vi "Static Read.vi"(8 "error in (no error)":errorcluster, 11 "Abs_I16 Integer in":refnum<class "Abs_I16 Integer.lvclass">) -> (0 "error out":errorcluster, 2 "Value":i16, 3 "Abs_I16 Integer out":refnum<class "Abs_I16 Integer.lvclass">)   [LabVIEW 2021, in "Abs_I16 Integer.lvclass"]
uses:
  Abs_I16 Integer.lvclass
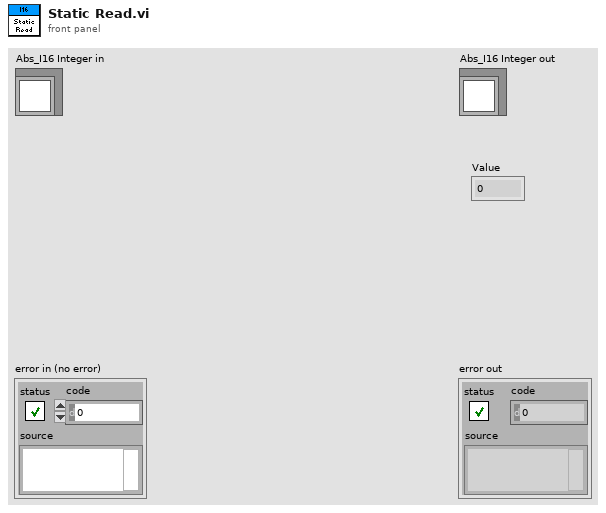
[diagram p1: front panel]
types:
  T1 = typedef "Abs_I16 Integer.lvclass/Type.ctl" = i16
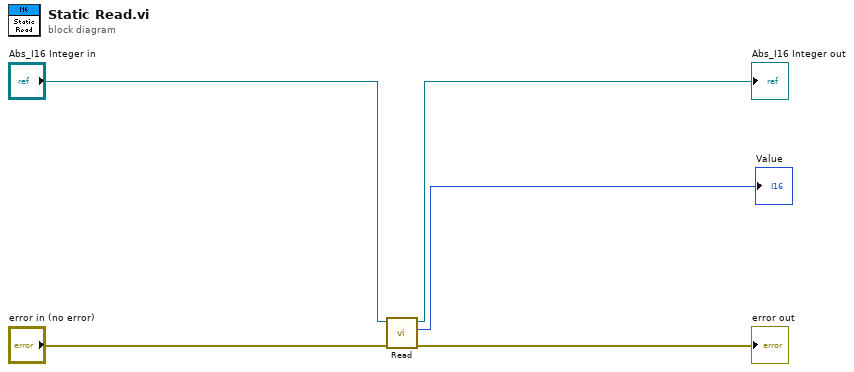
[diagram p0: block diagram]
diagram:
  n1 = call-dynamic "Read.vi"("error in (no error)"="error in (no error)", "Double Float.lvclass_340760 in"="Abs_I16 Integer in") -> ("error out"=→"error out":errorcluster, "Value"=→"Value":T1, "Double Float.lvclass_340760 out"=→"Abs_I16 Integer out":refnum<class "Abs_I16 Integer.lvclass">)  [unwired: 7 in]
